vi "Error Query.vi"(8 "error in (no error)":errorcluster, 11 "VISA resource name":refnum<visa-resource-name>) -> (0 "error out":errorcluster, 1 "Error Message":string, 2 "Error Code":i32[](array[numeric]), 3 "VISA resource name out":refnum<visa-resource-name>)   [LabVIEW 2016, in "Keithley 2450.lvlib"]
doc: "Queries the instrument for any errors in the instrument's error queue. It will continue to read errors until all errors have been read from the instrument. Any errors will be returned in the <B>error out</B> control.\n\nNote:\nThis VI is called automatically by most driver VIs so it is not usually necessary to call this in an application."
uses:
  Keithley 2450.lvlib
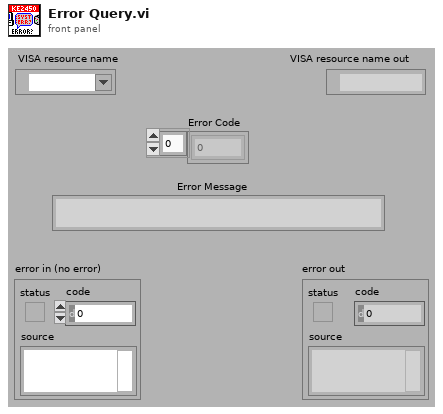
[diagram p1: front panel]
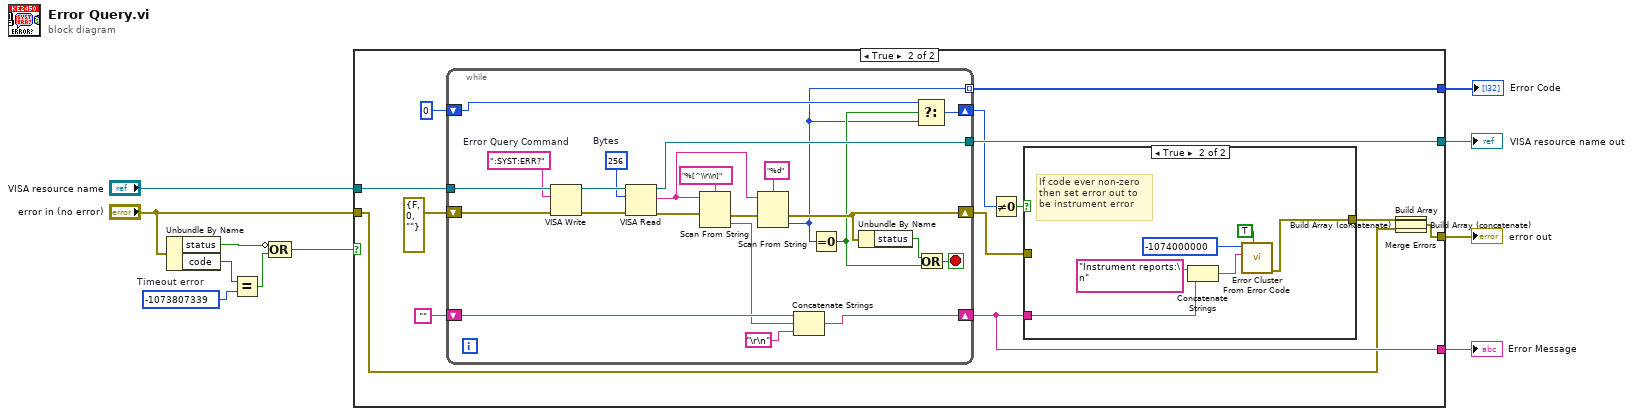
[diagram p0: block diagram]
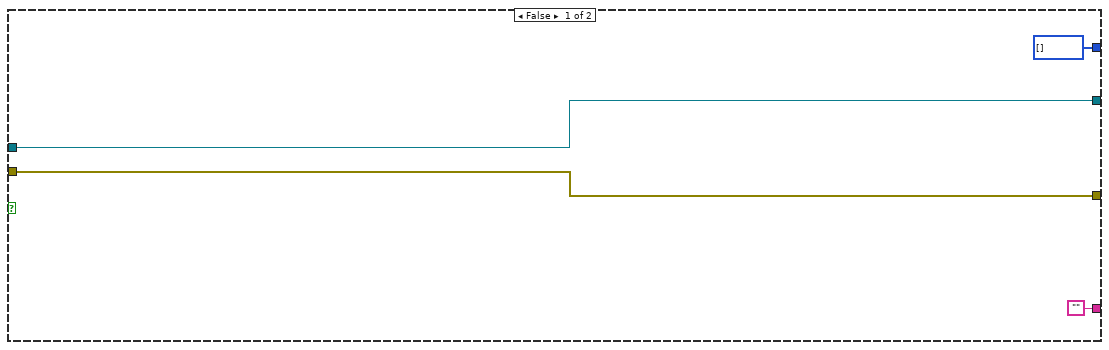
[diagram p2: hidden frame]
diagram:
  w6 = -1073807339  # Timeout error
  n1 = Unbundle By Name("error in (no error)") -> ("status"=w7:bool, "code"=w4:i32)
  n2 = Equal?(x=w4, y=w6) -> (x = y?=w5:bool)
  n3 = Compound Arithmetic op=OR(invert w7, w5) -> (w3:bool)
  n4 = case shown="True" w3 {
    tunnel: [w15 w31] -> w11
    tunnel: "VISA resource name" -> [w15 w30]
    tunnel: "error in (no error)" -> [w14 w20]
    tunnel: [w14 w28] -> w9
    tunnel: ["" w22] -> w2
    tunnel: [i32[] [] w21] -> w1
    frame False {
    }
    frame True {
      n5 = while {
        tunnel: [w61] -> w31
        tunnel: w30 -> [w60]
        shift-right: [w48] -> w22
        shift-left: "" -> [w51]
        shift-right: [w46] -> w23
        shift-left: 0 -> [w47]
        shift-right: [w44] -> w19
        shift-left: errorcluster {"status"=FALSE, "code"=0, "source"=""} ("error in (no error)") -> [w45]
        tunnel: [w39] -> w21 mode=indexing
        stop <- w54 stop-if-true
        w58 = u32 256  # Bytes
        w56 = ":SYST:ERR?"  # Error Query Command
        n6 = VISA Write(VISA resource name=w60, write buffer=w56, error in (no error)=w45) -> (VISA resource name out=w59:refnum<visa-resource-name>, error out=w57:errorcluster)  [unwired: 1 out]
        n7 = VISA Read(VISA resource name=w59, byte count=w58, error in (no error)=w57) -> (VISA resource name out=w61:refnum<visa-resource-name>, read buffer=w52:string, error out=w43:errorcluster)  [unwired: 1 out]
        n8 = Scan From String(format string="%[^\\r\\n]", input string=w52, error in=w43) -> (error out=w42:errorcluster, output 1=w49:string)  [unwired: 1 in, 3 out]
        n9 = Scan From String(format string="%d", input string=w52, error in=w42) -> (error out=w44:errorcluster, output 1=w39:i32)  [unwired: 1 in, 3 out]
        n10 = Concatenate Strings(w51, w49, "\r\n") -> (w48:string)
        n11 = Equal To 0?(x=w39) -> (x = 0?=w40:bool)
        n12 = Unbundle By Name(w44) -> ("status"=w41:bool)
        n13 = Select(t=w47, s=w40, f=w39) -> (s? t:f=w46:i32)
        n14 = Or(x=w41, y=w40) -> (x .or. y?=w54:bool)
      }
      n15 = Not Equal To 0?(x=w23) -> (x != 0?=w26:bool)
      n16 = case shown="True" w26 {
        tunnel: w22 -> [_ w37]
        tunnel: [w32 w33] -> w25
        tunnel: w19 -> [w32 _]
        frame False {
        }
        frame True {
          # "If code ever non-zero\nthen set error out to\nbe instrument error"
          n17 = Concatenate Strings("Instrument reports:\n" ("Source"), w37) -> (w34:string)
          n18 = call <vilib>:"Error Cluster From Error Code.vi"("show call chain? (False)"=TRUE, "error message (\"\")"=w34, "error code (0)"=-1074000000 ("Code")) -> ("error out"=w33:errorcluster)  [unwired: 1 in, 5 out]
        }
      }
      n19 = Build Array(w25, w20) -> (w18:errorcluster[])
      n20 = Build Array (concatenate)(w18) -> (w17:errorcluster[])
      n21 = Build Array (concatenate)(w17) -> (w16:errorcluster[])
      n22 = Merge Errors(w16) -> (w28:errorcluster)
    }
  }
  "VISA resource name out" <- w11
  "error out" <- w9
  "Error Message" <- w2
  "Error Code" <- w1
